vi "Get PWM Configuration.vi"(8 "error in":errorcluster, 10 "channels":refnum<class "Channel.lvclass">[](array[class]), 11 "PWM Mode in":refnum<class "PWM Mode.lvclass">) -> (0 "error out":errorcluster, 2 "PWM":T1 {"PWM Channels"."PWM frequency" items=["1 Hz", "50 Hz", "250 Hz", "500 Hz", "1 kHz", "5 kHz", "10 kHz", "20 kHz"]}, 3 "PWM Mode out":refnum<class "PWM Mode.lvclass">)   [LabVIEW 2017, in "Scan Engine Scripting.lvlib" / "PWM Mode.lvclass"]
uses:
  PWM Mode.lvclass
  Channel Classes/Channel/Channel.lvclass
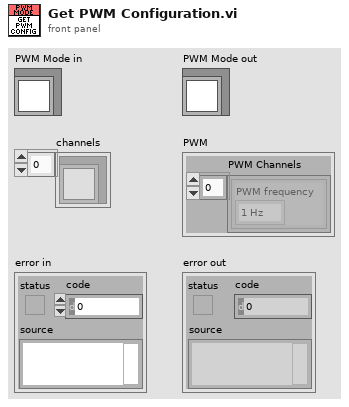
[diagram p1: front panel]
types:
  T1 = cluster{"PWM Channels":cluster{"PWM frequency":u32}[]}
  T2 = typedef "Scan Engine Scripting.lvlib/pwm channel settings.ctl" = cluster{"name":string, "default value":dbl, "frequency":T3}
  T3 = typedef "Scan Engine Scripting.lvlib/PWM Output Channel.lvclass/Frequency.ctl" = enum16{"1 Hz (1,000,000 us)", "50 Hz (20,000 us)", "250 Hz (4,000 us)", "500 Hz (2,000 us)", "1 kHz (1,000 us)", "5 kHz (200 us)", "10 kHz (100 us)", "20 kHz (50 us)"}
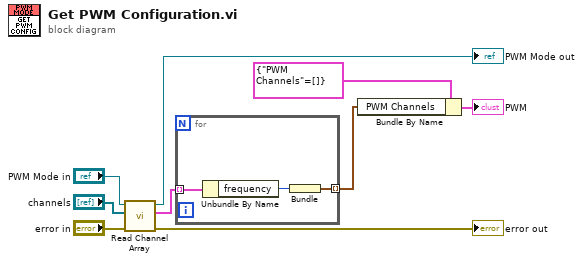
[diagram p0: block diagram]
diagram:
  n1 = call "Read Channel Array.vi"("error in"="error in", "channels"="channels", "digital output mode in"="PWM Mode in") -> ("error out"=→"error out":errorcluster, "channel settings"=w4:T2[], "digital output mode out"=→"PWM Mode out":refnum<class "PWM Mode.lvclass">)  [unwired: 6 in]
  n2 = for {
    tunnel: w4 -> [w12] mode=indexing
    tunnel: [w10] -> w2 mode=indexing
    n3 = Unbundle By Name(w12) -> ("frequency"=w11:T3)
    n4 = Bundle("frequency"=w11) -> (w10:cluster{"frequency":T3})  [unwired: 1 in]
  }
  n5 = Bundle By Name(cluster=T1 {"PWM Channels"=[]} ("PWM"), "PWM Channels"=w2) -> (→"PWM":T1)
